vi "Begin.vi"(8 "error in":errorcluster) -> (0 "error out":errorcluster)   [LabVIEW 2016]
doc: "Called before other user functions, this VI is expected to open initial I/O refnums, load in file data, and do all program initialization. Notice that the <B>error out</B> terminal is simply used for data flow. Wiring it to other structures or subVIs ensures that this VI runs first."
uses:
  <vilib>/Rock Robotics/WPI/DriverStation/WPI_DriverStationRobotMode2.ctl
  <vilib>/Rock Robotics/WPI/SafetyOutput/WPI_SafetyOutputConfigMenu.ctl
  <vilib>/Rock Robotics/WPI/Joystick/WPI_JoystickDeviceEnum.ctl
  <vilib>/Rock Robotics/SystemInterfaces/DIO/FPGA_DIOPWMChannel.ctl
  <vilib>/Rock Robotics/WPI/Solenoid/WPI_SolenoidChannel.ctl
  <vilib>/Rock Robotics/SystemInterfaces/DIO/FPGA_DIORelayChannel.ctl
  Robot Global Data.vi
  <vilib>/Rock Robotics/Network Tables/NT Write String Array.vi
  <vilib>/Rock Robotics/WPI/RobotDrive/WPI_RobotDriveOpen4MotorWithTalon.vi
  <vilib>/Rock Robotics/WPI/Solenoid/WPI_SolenoidOpenDouble.vi
  <vilib>/Rock Robotics/WPI/Utilities/WPI_GetSetVariantRefNum.vi
  <vilib>/Rock Robotics/WPI/Solenoid/WPI_SolenoidOpenSingle.vi
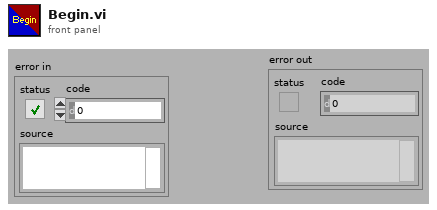
[diagram p1: front panel]
types:
  T1 = typedef "WPI_SolenoidChannel.ctl" = enum8{"Solenoid 0", "Solenoid 1", "Solenoid 2", "Solenoid 3", "Solenoid 4", "Solenoid 5", "Solenoid 6", "Solenoid 7", "Invalid"}
  T2 = typedef "FPGA_DIORelayChannel.ctl" = enum8{"Relay 0", "Relay 1", "Relay 2", "Relay 3", "Invalid"}
  T3 = typedef "WPI_JoystickDeviceEnum.ctl" = enum16{"USB 0", "USB 1", "USB 2", "USB 3", "USB 4", "USB 5"}
  T4 = typedef "FPGA_DIOPWMChannel.ctl" = enum8{"PWM 0", "PWM 1", "PWM 2", "PWM 3", "PWM 4", "PWM 5", "PWM 6", "PWM 7", "PWM 8", "PWM 9", "PWM MXP 0", "PWM MXP 1", "PWM MXP 2", "PWM MXP 3", "PWM MXP 4", "PWM MXP 5", "PWM MXP 6", "PWM MXP 7", "PWM MXP 8", "PWM MXP 9", "Invalid"}
  T5 = typedef "WPI_SafetyOutputConfigMenu.ctl" = enum16{"Enable", "Disable"}
  T6 = typedef "WPI_DriverStationRobotMode2.ctl" = enum16{"Autonomous Disabled", "Autonomous Enabled", "Teleop Disabled", "Teleop Enabled", "Disconnected", "Finish", "Test Disabled", "Test Enabled", "Emergency Stopped"}
  T7 = typedef "WPI_RelayDevRef.ctl" = cluster{"DevStatus":errorcluster, "Relay Channel":T2, "Relay Direction":T8}
  T8 = typedef "WPI_RelayDirection.ctl" = enum16{"Both directions", "Forward only", "Reverse only"}
  T9 = typedef "WPI_CompressorDevRef.ctl" = cluster{"DevStatus":errorcluster, "Pneumatics Control Module":u8}
  T10 = typedef "WPI_MotorControlDeviceRef.ctl" = cluster{"DeviceStatus":errorcluster, "Type":T11, "PWM":cluster{"PWM Channel":T4, "DeadBand":T12}, "CAN":cluster{"Device Number":u8, "SetOutput VI Ref":variant, "GetOutput VI Ref":variant, "Enable VI Ref":variant, "Disable VI Ref":variant, "Data":variant}, "Invert":bool}
  T11 = typedef "WPI_MotorControlType.ctl" = enum16{"PWM", "CAN"}
  T12 = typedef "WPI_PWMDeadband.ctl" = cluster{"Name":string, "maxPositivePwm":i32, "minPositivePwm":i32, "centerPwm":i32, "maxNegativePwm":i32, "minNegativePwm":i32, "angularRange":u16}
  T13 = typedef "WPI_JoystickDevRef.ctl" = cluster{"Device":T3}
  T14 = typedef "WPI_RobotDriveDevRef.ctl" = cluster{"DevStatus":errorcluster, "Motors[]":T10[], "Square Inputs":bool, "Max Output":dbl}
  T15 = typedef "WPI_SolenoidDevRef.ctl" = cluster{"DevStatus":errorcluster, "Pneumatics Control Module":u8, "Forward Solenoid Channel":T1, "Reverse Solenoid Channel":T1}
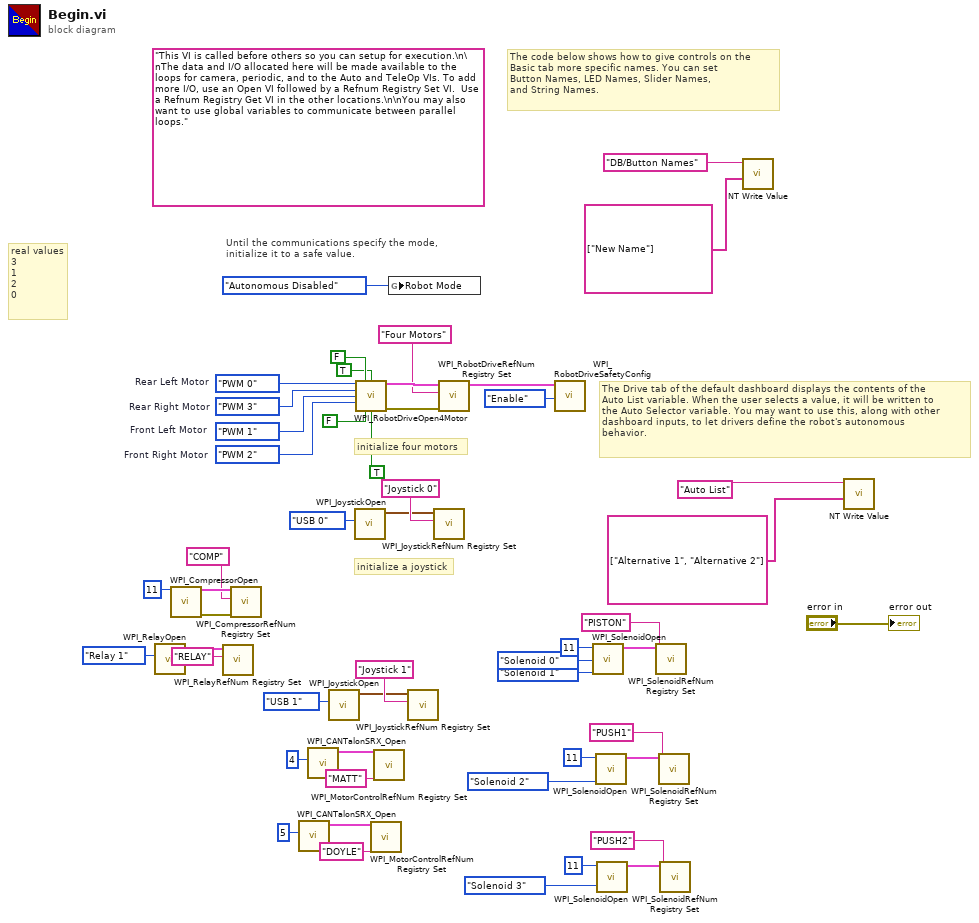
[diagram p0: block diagram]
diagram:
  w34 = FPGA_DIOPWMChannel."PWM 2"  # Front Right Motor
  w35 = FPGA_DIOPWMChannel."PWM 1"  # Front Left Motor
  w36 = FPGA_DIOPWMChannel."PWM 3"  # Rear Right Motor
  w37 = FPGA_DIOPWMChannel."PWM 0"  # Rear Left Motor
  (unwired) "This VI is called before others so you can setup for execution.\n\nThe data and I/O allocated here will be made available to the loops for camera, periodic, and to the Auto and TeleOp VIs. To add more I/O, use an Open VI followed by a Refnum Registry Set VI.  Use a Refnum Registry Get VI in the other locations.\n\nYou may also want to use global variables to communicate between parallel loops."
  # "real values\n3\n1\n2\n0"
  # "initialize a joystick"
  # "initialize four motors"
  # "The Drive tab of the default dashboard displays the contents of the\nAuto List variable. When the user selects a value, it will be written to\nthe Auto Selector variable. You may want to use this, along with other\ndashboard inputs, to let drivers define the robot's autonomous\nbehavior."
  # "The code below shows how to give controls on the\nBasic tab more specific names. You can set\nButton Names, LED Names, Slider Names,\nand String Names."
  # "Until the communications specify the mode,\ninitialize it to a safe value."
  n1 = call <vilib>:"WPI_RelayOpen.vi"("Relay Channel"=FPGA_DIORelayChannel."Relay 1") -> ("RelayDevRef"=w21:T7)  [unwired: 9 in, 1 out]
  n2 = call <vilib>:"WPI_CompressorOpen.vi"("Pneumatics Control Module (0)"=u8 11) -> ("CompressorDevRef"=w11:T9, "error out"=w12:errorcluster)  [unwired: 13 in]
  n3 = call <vilib>:"WPI_RelayRefNum Registry Set.vi"("refnum name"="RELAY", "RelayDevRef"=w21) -> ()  [unwired: 8 in, 2 out]
  n4 = call <vilib>:"WPI_CompressorRefNum Registry Set.vi"("error in (no error)"=w12, "refnum name"="COMP", "CompressorDevRef"=w11) -> ()  [unwired: 7 in, 2 out]
  n5 = call <vilib>:"WPI_CANTalonSRX_Open.vi"("Device Number"=u8 5) -> ("CAN Talon SRX Ref"=w17:T10)  [unwired: 9 in, 1 out]
  n6 = call <vilib>:"WPI_CANTalonSRX_Open.vi"("Device Number"=u8 4) -> ("CAN Talon SRX Ref"=w18:T10)  [unwired: 9 in, 1 out]
  n7 = call <vilib>:"WPI_JoystickOpen.vi"("JoystickDevice"=WPI_JoystickDeviceEnum."USB 1") -> ("JoystickDevRef"=w32:T13)  [unwired: 10 in]
  n8 = call <vilib>:"WPI_JoystickOpen.vi"("JoystickDevice"=WPI_JoystickDeviceEnum."USB 0") -> ("JoystickDevRef"=w39:T13)  [unwired: 10 in]
  n9 = call-poly <vilib>:"WPI_RobotDriveOpen4Motor.vi"("Rear Left Motor"=w37, "Rear Left Motor Inverted"=FALSE, "Rear Right Motor Inverted"=TRUE, "Rear Right Motor"=w36, "Front Left Motor"=w35, "Front Right Motor"=w34, "Front Left Motor Inverted"=FALSE, "Front Right Motor Inverted"=TRUE) -> ("RobotDriveDevRef"=w45:T14, "error out"=w43:errorcluster)  [unwired: 6 in]
  n10 = call <vilib>:"WPI_MotorControlRefNum Registry Set.vi"("refnum name"="DOYLE", "MotorControlDevRef"=w17) -> ()  [unwired: 8 in, 2 out]
  n11 = call <vilib>:"WPI_MotorControlRefNum Registry Set.vi"("refnum name"="MATT", "MotorControlDevRef"=w18) -> ()  [unwired: 8 in, 2 out]
  n12 = global write "Robot Global Data.vi" "Robot Mode"(WPI_DriverStationRobotMode2."Autonomous Disabled" ("Robot Mode")) -> ()
  n13 = call <vilib>:"WPI_JoystickRefNum Registry Set.vi"("refnum name"="Joystick 1", "JoystickDevRef"=w32) -> ()  [unwired: 8 in, 2 out]
  n14 = call <vilib>:"WPI_JoystickRefNum Registry Set.vi"("refnum name"="Joystick 0", "JoystickDevRef"=w39) -> ()  [unwired: 8 in, 2 out]
  n15 = call <vilib>:"WPI_RobotDriveRefNum Registry Set.vi"("error in (no error)"=w43, "refnum name"="Four Motors", "RobotDriveDevRef"=w45) -> ("RobotDriveDevRef"=w42:T14)  [unwired: 1 in, 7 out]
  n16 = call <vilib>:"WPI_RobotDriveSafetyConfig.vi"("mode"=WPI_SafetyOutputConfigMenu."Enable", "RobotDriveDevRef"=w42) -> ()  [unwired: 8 in, 2 out]
  n17 = call-poly <vilib>:"WPI_SolenoidOpen.vi"("Reverse Solenoid Channel"=WPI_SolenoidChannel."Solenoid 1", "Forward Solenoid Channel"=WPI_SolenoidChannel."Solenoid 0", "Pneumatics Control Module (0)"=u8 11) -> ("SolenoidDevRef"=w23:T15)  [unwired: 7 in, 1 out]
  n18 = call-poly <vilib>:"WPI_SolenoidOpen.vi"("Solenoid Channel"=WPI_SolenoidChannel."Solenoid 2" ("Forward Solenoid Channel"), "Pneumatics Control Module (0)"=u8 11) -> ("SolenoidDevRef"=w7:T15)  [unwired: 8 in, 1 out]
  n19 = call-poly <vilib>:"WPI_SolenoidOpen.vi"("Solenoid Channel"=WPI_SolenoidChannel."Solenoid 3" ("Forward Solenoid Channel"), "Pneumatics Control Module (0)"=u8 11) -> ("SolenoidDevRef"=w2:T15)  [unwired: 8 in, 1 out]
  n20 = call <vilib>:"WPI_SolenoidRefNum Registry Set.vi"("refnum name"="PISTON", "SolenoidDevRef"=w23) -> ()  [unwired: 8 in, 2 out]
  n21 = call <vilib>:"WPI_SolenoidRefNum Registry Set.vi"("refnum name"="PUSH1", "SolenoidDevRef"=w7) -> ()  [unwired: 8 in, 2 out]
  n22 = call <vilib>:"WPI_SolenoidRefNum Registry Set.vi"("refnum name"="PUSH2", "SolenoidDevRef"=w2) -> ()  [unwired: 8 in, 2 out]
  n23 = call-poly <vilib>:"NT Write Value.vi"("String Array"=string[] ["New Name"], "Name"="DB/Button Names") -> ()  [unwired: 9 in, 1 out]
  n24 = call-poly <vilib>:"NT Write Value.vi"("String Array"=string[] ["Alternative 1", "Alternative 2"], "Name"="Auto List") -> ()  [unwired: 9 in, 1 out]
  "error out" <- "error in"
